vi "LOERN_GetAutoToolRegions.vi"(0 "XRef":T9, 1 "State In":T7={"Inputs"=1, "SelectedIndex"=0, "ClassInfo"=[]}) -> (14 "Regions":T2, 15 "Fatal Error Out":T1)   [LabVIEW 2016, in "LV Object Event Registration Node.xnode"]
uses:
  LV Object Event Registration Node.xnode
  <vilib>/XNodeSupport/XNodeXNodeRef.ctl
  LOERN_State.ctl
  LOERN_ClassInfo.ctl
  <vilib>/XNodeSupport/XNodeAutotoolRegions.ctl
  <vilib>/XNodeSupport/XNodeAutotoolRegion.ctl
  <vilib>/XNodeSupport/XNodeRect32.ctl
  <vilib>/XNodeSupport/XNodeInt.ctl
  <vilib>/XNodeSupport/XNodeTools.ctl
  <vilib>/XNodeSupport/XNodeErrorCluster.ctl
  <vilib>/XNodeSupport/NI_XNodeSupport.lvlib
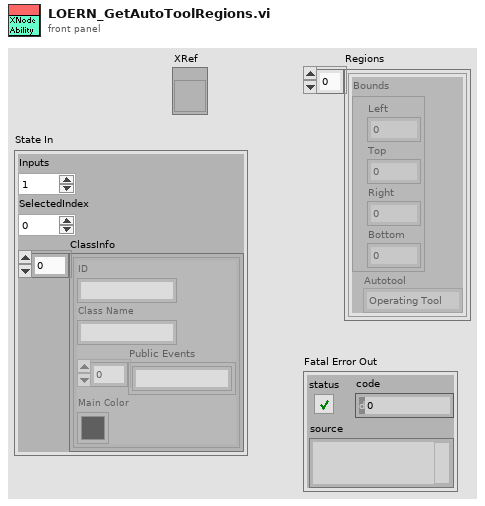
[diagram p1: front panel]
types:
  T1 = typedef "NI_XNodeSupport.lvlib/XNodeErrorCluster.ctl" = errorcluster
  T2 = typedef "NI_XNodeSupport.lvlib/XNodeAutotoolRegions.ctl" = T3[]
  T3 = typedef "NI_XNodeSupport.lvlib/XNodeAutotoolRegion.ctl" = cluster{"Bounds":T4, "Autotool":T6}
  T4 = typedef "NI_XNodeSupport.lvlib/XNodeRect32.ctl" = cluster{"Left":T5, "Top":T5, "Right":T5, "Bottom":T5}
  T5 = typedef "NI_XNodeSupport.lvlib/XNodeInt.ctl" = i32
  T6 = typedef "NI_XNodeSupport.lvlib/XNodeTools.ctl" = enum32{"Operating Tool", "Placement Tool", "Labelling Tool", "Wiring Tool", "Scroll Tool", "Breakpoint Tool", "Probe Tool", "Auto Tool"}
  T7 = typedef "LV Object Event Registration Node.xnode/LOERN_State.ctl" = cluster{"Inputs":u16, "SelectedIndex":i16, "ClassInfo":T8[]}
  T8 = typedef "LV Object Event Registration Node.xnode/LOERN_ClassInfo.ctl" = cluster{"ID":string, "Class Name":string, "Public Events":string[], "Main Color":u32}
  T9 = typedef "NI_XNodeSupport.lvlib/XNodeXNodeRef.ctl" = refnum<vi>
  T10 = typedef "NI_XNodeSupport.lvlib/XNodeBounds.ctl" = cluster{"Width":T5, "Height":T5}
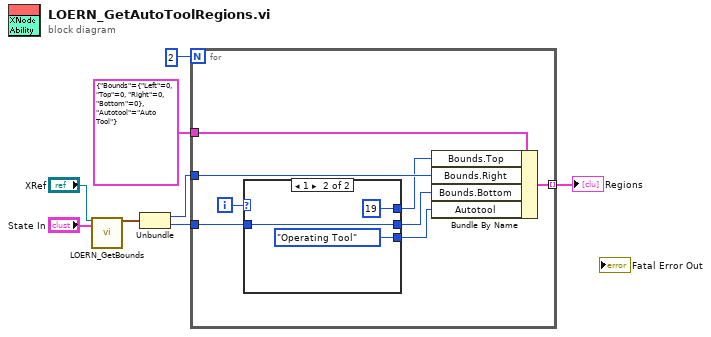
[diagram p0: block diagram]
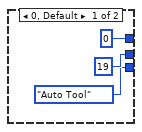
[diagram p2: hidden frame]
diagram:
  n1 = call "LOERN_GetBounds.vi"("XRef"="XRef", "State In"="State In") -> ("Bounds"=w6:T10)  [unwired: 16 in, 1 out]
  n2 = Unbundle(w6) -> ("Width"=w3:T5, "Height"=w2:T5)
  n3 = for {
    N: 2 -> [_]
    tunnel: T3 {"Bounds"={"Left"=0, "Top"=0, "Right"=0, "Bottom"=0}, "Autotool"=enum."Auto Tool"} ("Autotool Region") -> [w16]
    tunnel: w3 -> [w14]
    tunnel: w2 -> [w10]
    tunnel: [w9] -> w1 mode=indexing
    i -> [w15]
    n4 = case shown="1" w15 {
      tunnel: [0 19] -> w13
      tunnel: [19 w20] -> w12
      tunnel: [XNodeTools."Auto Tool" ("Autotool") XNodeTools."Operating Tool" ("Autotool")] -> w11
      tunnel: w10 -> [_ w20]
      frame 0, Default {
      }
      frame 1 {
      }
    }
    n5 = Bundle By Name(cluster=w16, "Bounds.Top"=w13, "Bounds.Right"=w14, "Bounds.Bottom"=w12, "Autotool"=w11) -> (w9:T3)
  }
  "Regions" <- w1
